vi "claw work 2.vi"   [LabVIEW 2010, in "ClawBot.lvrbt"]
uses:
  ClawBot.lvrbt
  <vilib>/NXT/Block Support/NXT_InputPort.ctl
  <vilib>/NXT/Subs/MotorOutput.ctl
  <vilib>/NXT/Dual Mode Library/Sensors/Touch_Pressed.vi
types:
  T1 = typedef "NXT_InputPort.ctl" = u8
  T2 = typedef "MotorOutput.ctl" = u8
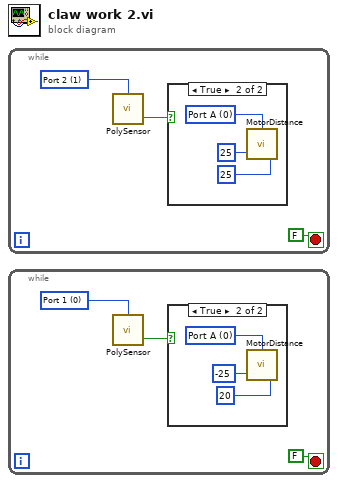
[diagram p0: block diagram]
diagram:
  n1 = while {
    stop <- FALSE stop-if-true
    w2 = T1 1 items=["Port 1", "Port 2", "Port 3", "Port 4"] ("Port (Port 1)")
    n2 = call-poly <vilib>:"PolySensor.vi"("Port (Port 1)"=w2) -> ("Yes / No"=w3:bool)  [unwired: 2 in, 1 out]
    n3 = case shown="True" w3 {
      frame False {
      }
      frame True {
        w6 = T2 0 items=["Port A"=0, "Port B"=1, "Port C"=2, "Ports A & B"=4, "Ports A & C"=5, "Ports B & C"=6, "All Ports"=3] ("Output Port (All Ports)")
        n4 = call <vilib>:"MotorDistance.vi"("Power (75)"=25, "Angle of Rotation (360)"=25, "Output Port (All Ports)"=w6) -> ()  [unwired: 1 in, 1 out]
      }
    }
  }
  n5 = while {
    stop <- FALSE stop-if-true
    w9 = T1 0 items=["Port 1", "Port 2", "Port 3", "Port 4"] ("Port (Port 1)")
    n6 = call-poly <vilib>:"PolySensor.vi"("Port (Port 1)"=w9) -> ("Yes / No"=w7:bool)  [unwired: 2 in, 1 out]
    n7 = case shown="True" w7 {
      frame False {
      }
      frame True {
        w12 = T2 0 items=["Port A"=0, "Port B"=1, "Port C"=2, "Ports A & B"=4, "Ports A & C"=5, "Ports B & C"=6, "All Ports"=3] ("Output Port (All Ports)")
        n8 = call <vilib>:"MotorDistance.vi"("Power (75)"=-25, "Angle of Rotation (360)"=20, "Output Port (All Ports)"=w12) -> ()  [unwired: 1 in, 1 out]
      }
    }
  }
